vi "Create Directory for Dependency.vi"(0 "directory path":path, 11 "error in":errorcluster) -> (4 "directory path out":path, 15 "error out":errorcluster)   [LabVIEW 2021, in "Multiple Converter.lvlib"]
uses:
  Multiple Converter.lvlib
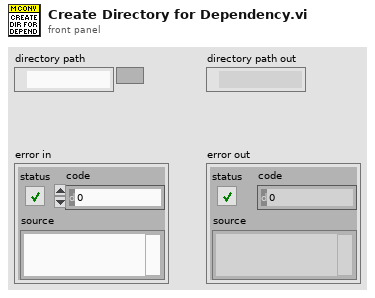
[diagram p1: front panel]
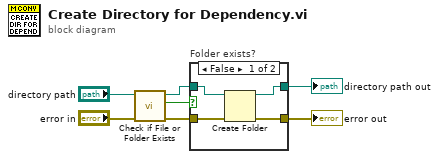
[diagram p0: block diagram]
diagram:
  n1 = call <vilib>:"Check if File or Folder Exists.vi"("error in (no error)"="error in", "path"="directory path") -> ("error out"=w3:errorcluster, "file or folder exists?"=w2:bool, "dup path"=w6:path)  [unwired: 7 in]
  n2 = case "Folder exists?" shown="False" w2 {
    tunnel: w3 -> [w11 w13]
    tunnel: [w10 w13] -> w4
    tunnel: w6 -> [w9 w12]
    tunnel: [w8 w12] -> w1
    frame False {
      n3 = Create Folder(path (use dialog)=w9, error in=w11) -> (created path=w8:path, error out=w10:errorcluster)  [unwired: 1 in, 1 out]
    }
    frame True {
    }
  }
  "error out" <- w4
  "directory path out" <- w1
